vi "Time Stamp 64 to LabVIEW Time Stamp.vi"(8 "Error In":errorcluster, 11 "Time Stamp 64":T1) -> (0 "Error Out":errorcluster, 3 "LabVIEW Time Stamp":timestamp)   [LabVIEW 2021, in "SNTP.lvlib"]
uses:
  SNTP.lvlib
  Public/Controls/Time Stamp 64.ctl
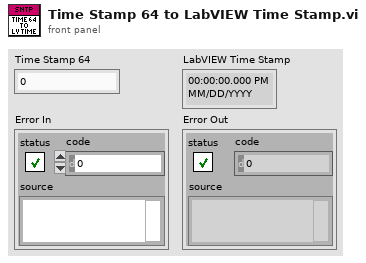
[diagram p1: front panel]
types:
  T1 = typedef "SNTP.lvlib/Time Stamp 64.ctl" = fxp<+,64,32>
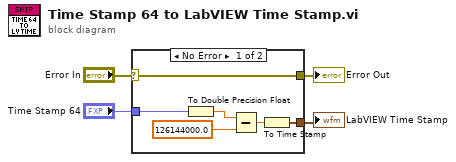
[diagram p0: block diagram]
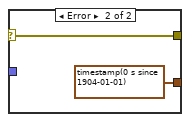
[diagram p2: hidden frame]
diagram:
  n1 = case shown="No Error" "Error In" {
    selector: "Error In" -> [w10 w12]
    tunnel: [w10 w12] -> w3
    tunnel: "Time Stamp 64" -> [w6 _]
    tunnel: [w5 timestamp(0 s since 1904-01-01)] -> w1
    frame No Error {
      n2 = To Double Precision Float(number=w6) -> (double precision float=w8:dbl)
      n3 = Subtract(x=w8, y=126144000.0) -> (x-y=w9:dbl)
      n4 = To Time Stamp(1:w9) -> (0:w5:timestamp)
    }
    frame Error {
    }
  }
  "LabVIEW Time Stamp" <- w1
  "Error Out" <- w3
